vi "CSVImport_WhileLoop_Iter.vi"() -> ()   [LabVIEW 2021]
uses:
  <vilib>/Utility/file.llb/Read Delimited Spreadsheet (DBL).vi
panel:
  out "Array":dbl[](array[numeric])
  out "OUTPUT":dbl
  out "Phase II Iterations":i32
  in  "TickLength":u32
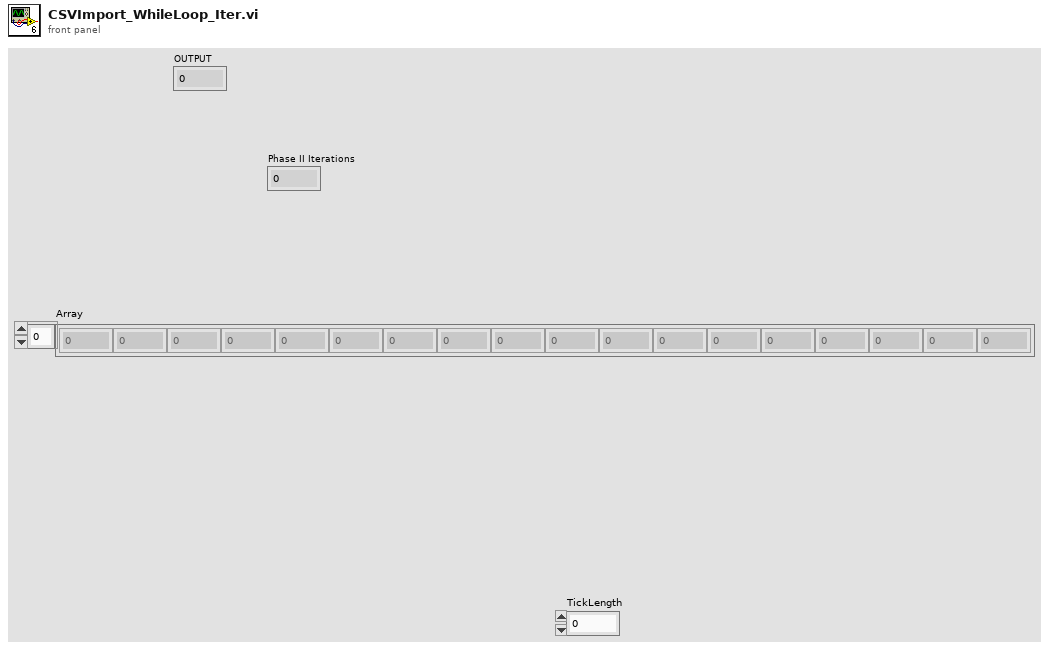
[diagram p1: front panel]
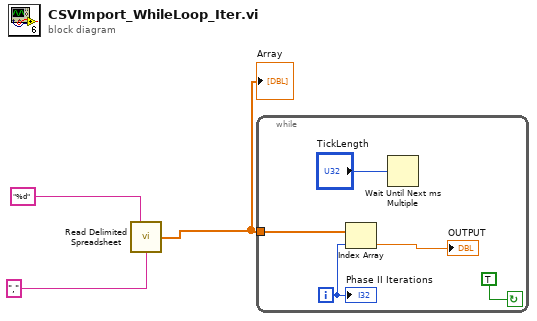
[diagram p0: block diagram]
diagram:
  n1 = call-poly <vilib>:"Read Delimited Spreadsheet.vi"("format (%.3f)"="%d", "delimiter (\\t)"=",") -> ("first row"=w1:dbl[])  [unwired: 8 in, 5 out]
  "Array" <- w1
  n2 = while {
    tunnel: w1 -> [w6]
    i -> [w4]
    stop <- TRUE continue-if-true
    n3 = Index Array "Index Array"(array=w6, index=w4) -> (element=→"OUTPUT":dbl)
    n4 = Wait Until Next ms Multiple(millisecond multiple="TickLength") -> ()  [unwired: 1 out]
    "Phase II Iterations" <- w4
  }
